vi "manual arg compare key.vi"() -> (3 "manual key":string)   [LabVIEW 2016]
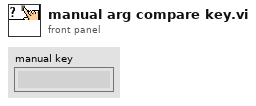
[diagram p1: front panel]
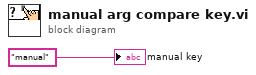
[diagram p0: block diagram]
diagram:
  "manual key" <- "manual" ("key")
